vi "Begin.vi"(8 "error in":errorcluster) -> (0 "error out":errorcluster)   [LabVIEW 2015]
doc: "Called before other user functions, this VI is expected to open initial I/O refnums, load in file data, and do all program initialization. Notice that the <B>error out</B> terminal is simply used for data flow. Wiring it to other structures or subVIs ensures that this VI runs first."
uses:
  <vilib>/Rock Robotics/WPI/DriverStation/WPI_DriverStationRobotMode2.ctl
  <vilib>/Rock Robotics/WPI/Joystick/WPI_JoystickDeviceEnum.ctl
  <vilib>/Rock Robotics/WPI/Solenoid/WPI_SolenoidChannel.ctl
  <vilib>/Rock Robotics/SystemInterfaces/DIO/FPGA_DIOPWMChannel.ctl
  <vilib>/Rock Robotics/WPI/SafetyOutput/WPI_SafetyOutputConfigMenu.ctl
  <vilib>/Rock Robotics/SystemInterfaces/DIO/FPGA_DIOChannel.ctl
  Robot Global Data.vi
  <vilib>/Rock Robotics/Network Tables/NT Write String Array.vi
  <vilib>/Rock Robotics/WPI/Solenoid/WPI_SolenoidOpenSingle.vi
  <vilib>/Rock Robotics/WPI/MotorControl/WPI_MotorControlOpen Talon.vi
  <vilib>/Rock Robotics/WPI/MotorControl/WPI_MotorControlOpenCANTalonSRX.vi
  <vilib>/Rock Robotics/WPI/RobotDrive/WPI_RobotDriveOpen4MotorWithCANTalonSRX.vi
  <vilib>/Rock Robotics/WPI/Counter/WPI_CounterDigitalInputToDigitalSource.vi
  <vilib>/Rock Robotics/SystemInterfaces/AI/FPGA_AIGyroChannel.ctl
  <vilib>/Rock Robotics/WPI/MotorControl/WPI_MotorControlOpen Victor.vi
  <vilib>/Rock Robotics/WPI/Gyro/WPI_GyroAnalogOpen.vi
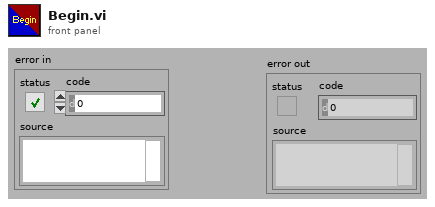
[diagram p1: front panel]
types:
  T1 = typedef "FPGA_DIOChannel.ctl" = enum8{"DIO 0", "DIO 1", "DIO 2", "DIO 3", "DIO 4", "DIO 5", "DIO 6", "DIO 7", "DIO 8", "DIO 9", "DIO MXP 0", "DIO MXP 1", "DIO MXP 2", "DIO MXP 3", "DIO MXP 4", "DIO MXP 5", "DIO MXP 6", "DIO MXP 7", "DIO MXP 8", "DIO MXP 9", "DIO MXP 10", "DIO MXP 11", "DIO MXP 12", "DIO MXP 13", "DIO MXP 14", "DIO MXP 15", "Invalid"}
  T2 = typedef "WPI_SafetyOutputConfigMenu.ctl" = enum16{"Enable", "Disable"}
  T3 = typedef "WPI_SolenoidChannel.ctl" = enum8{"Solenoid 0", "Solenoid 1", "Solenoid 2", "Solenoid 3", "Solenoid 4", "Solenoid 5", "Solenoid 6", "Solenoid 7", "Invalid"}
  T4 = typedef "FPGA_DIOPWMChannel.ctl" = enum8{"PWM 0", "PWM 1", "PWM 2", "PWM 3", "PWM 4", "PWM 5", "PWM 6", "PWM 7", "PWM 8", "PWM 9", "PWM MXP 0", "PWM MXP 1", "PWM MXP 2", "PWM MXP 3", "PWM MXP 4", "PWM MXP 5", "PWM MXP 6", "PWM MXP 7", "PWM MXP 8", "PWM MXP 9", "Invalid"}
  T5 = typedef "WPI_JoystickDeviceEnum.ctl" = enum16{"USB 0", "USB 1", "USB 2", "USB 3", "USB 4", "USB 5"}
  T6 = typedef "WPI_DriverStationRobotMode2.ctl" = enum16{"Autonomous Disabled", "Autonomous Enabled", "Teleop Disabled", "Teleop Enabled", "Disconnected", "Finish", "Test Disabled", "Test Enabled", "Emergency Stopped"}
  T7 = typedef "WPI_DigitalInputDevRef.ctl" = cluster{"DevStatus":errorcluster, "DIO Channel":T1}
  T8 = typedef "FPGA_CounterEncoderSourceConvertionLVSourceType.ctl" = cluster{"DevStatus":errorcluster, "AnalogTriggerMode?":bool, "DigitalMode":cluster{"DIO Channel":T9}, "AnalogTriggerMode":cluster{"AnalogTriggerIndex":T10, "OutputType":T11}}
  T9 = typedef "FPGA_DIODigitalSourceChannel.ctl" = enum8{"DIO 0", "DIO 1", "DIO 2", "DIO 3", "DIO 4", "DIO 5", "DIO 6", "DIO 7", "DIO 8", "DIO 9", "DIO MXP 0", "DIO MXP 1", "DIO MXP 2", "DIO MXP 3", "DIO MXP 4", "DIO MXP 5", "DIO MXP 6", "DIO MXP 7", "DIO MXP 8", "DIO MXP 9", "DIO MXP 10", "DIO MXP 11", "DIO MXP 12", "DIO MXP 13", "DIO MXP 14", "DIO MXP 15", "Disabled"}
  T10 = typedef "FPGA_AnalogTriggerIndex.ctl" = enum8{"Trig 0", "Trig 1", "Trig 2", "Trig 3", "Trig 4", "Trig 5", "Trig 6", "Trig 7", "Invalid"}
  T11 = typedef "FPGA_AnalogTriggerOutType.ctl" = enum16{"InWindow", "TriggerState", "Rising", "Falling"}
  T12 = typedef "WPI_EncoderDevRef.ctl" = cluster{"DevStatus":errorcluster, "EncoderIndex":T13, "CounterIndex":T14, "DistancePerCount":dbl, "Decoding Type":T15}
  T13 = typedef "FPGA_EncoderIdx.ctl" = enum8{"Enc 0", "Enc 1", "Enc 2", "Enc 3", "Enc 4", "Enc 5", "Enc 6", "Enc 7", "Invalid"}
  T14 = typedef "FPGA_CounterCtrSystemIndex.ctl" = enum8{"Ctr 0", "Ctr 1", "Ctr 2", "Ctr 3", "Ctr 4", "Ctr 5", "Ctr 6", "Ctr 7", "Invalid"}
  T15 = typedef "WPI_EncoderType.ctl" = enum16{"1x", "2x", "4x"}
  T16 = typedef "WPI_JoystickDevRef.ctl" = cluster{"Device":T5}
  T17 = typedef "WPI_SolenoidDevRef.ctl" = cluster{"DevStatus":errorcluster, "Pneumatics Control Module":u8, "Forward Solenoid Channel":T3, "Reverse Solenoid Channel":T3}
  T18 = typedef "WPI_MotorControlDeviceRef.ctl" = cluster{"DeviceStatus":errorcluster, "Type":T19, "PWM":cluster{"PWM Channel":T4, "DeadBand":T20}, "CAN":cluster{"Device Number":u8, "Control Mode":T21, "Semaphore":T22, "Max Vout":dbl, "TalonSRX Control Mode":T23}, "Invert":bool}
  T19 = typedef "WPI_MotorControlType.ctl" = enum16{"PWM", "CAN", "CANTalonSRX"}
  T20 = typedef "WPI_PWMDeadband.ctl" = cluster{"Name":string, "maxPositivePwm":i32, "minPositivePwm":i32, "centerPwm":i32, "maxNegativePwm":i32, "minNegativePwm":i32, "angularRange":u16}
  T21 = typedef "WPI_CANJaguar_ControlMode.ctl" = enum8{"Percent VBus", "Current", "Speed", "Position", "Voltage"}
  T22 = typedef "Semaphore RefNum" = refnum<k1>
  T23 = typedef "WPI_CANTalonSRX_APIControlMode.ctl" = enum8{"Percent VBus", "Speed", "Position", "Slave", "Unchanged / Invalid", "Voltage Compensation", "Current", "Motion Profile"}
  T24 = typedef "FPGA_AIGyroChannel.ctl" = enum8{"AI 0", "AI 1", "Invalid"}
  T25 = typedef "WPI_GyroDevRef.ctl" = cluster{"DevStatus":errorcluster, "Analog Channel":T26, "Offset":dbl, "Gain (VoltsPerDegree/Second)":dbl, "Gyro Type":enum16{"Analog", "XRS450"}, "Handle":i32, "SPI Bus":T27, "Device Found":bool, "Sample Rate":dbl, "Calibrate On Open":bool}
  T26 = typedef "FPGA_AIChannel.ctl" = enum8{"AI 0", "AI 1", "AI 2", "AI 3", "AI MXP 0", "AI MXP 1", "AI MXP 2", "AI MXP 3", "Invalid"}
  T27 = typedef "spi_bus.ctl" = enum16{"SPI On-Board, CS0", "SPI On-Board, CS1", "SPI On-Board, CS2", "SPI On-Board, CS3", "SPI MXP", "Invalid"}
  T28 = typedef "WPI_RobotDriveDevRef.ctl" = cluster{"DevStatus":errorcluster, "Motors[]":T18[], "Square Inputs":bool, "Max Output":dbl}
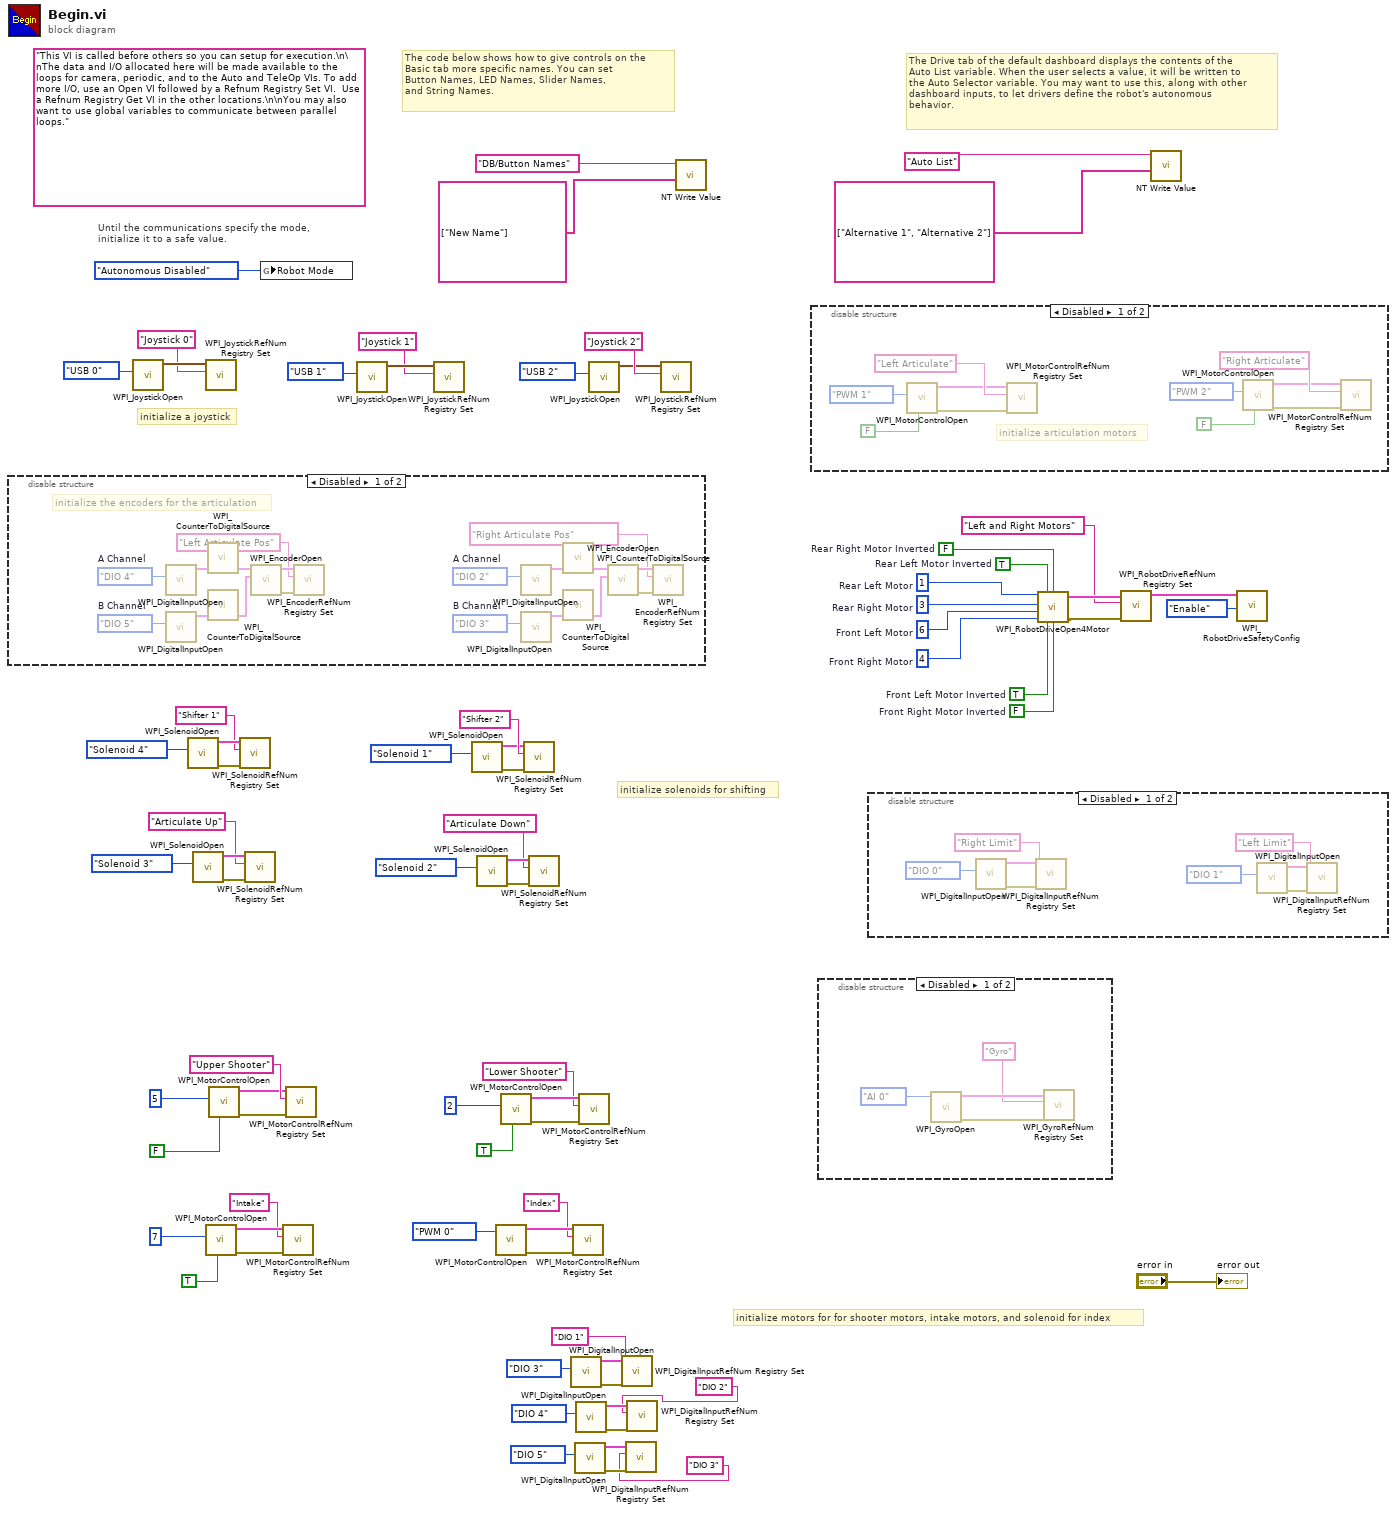
[diagram p0: block diagram]
diagram:
  w25 = u8 4  # Front Right Motor
  w24 = u8 3  # Rear Right Motor
  w23 = u8 6  # Front Left Motor
  w22 = u8 1  # Rear Left Motor
  w21 = TRUE  # Rear Left Motor Inverted
  w20 = FALSE  # Rear Right Motor Inverted
  w19 = FALSE  # Front Right Motor Inverted
  w18 = TRUE  # Front Left Motor Inverted
  (unwired) "This VI is called before others so you can setup for execution.\n\nThe data and I/O allocated here will be made available to the loops for camera, periodic, and to the Auto and TeleOp VIs. To add more I/O, use an Open VI followed by a Refnum Registry Set VI.  Use a Refnum Registry Get VI in the other locations.\n\nYou may also want to use global variables to communicate between parallel loops."
  # "initialize solenoids for shifting"
  # "initialize a joystick"
  # "initialize motors for for shooter motors, intake motors, and solenoid for index"
  # "The Drive tab of the default dashboard displays the contents of the\nAuto List variable. When the user selects a value, it will be written to\nthe Auto Selector variable. You may want to use this, along with other\ndashboard inputs, to let drivers define the robot's autonomous\nbehavior."
  # "The code below shows how to give controls on the\nBasic tab more specific names. You can set\nButton Names, LED Names, Slider Names,\nand String Names."
  # "Until the communications specify the mode,\ninitialize it to a safe value."
  n1 = disable-structure shown="Disabled" {
    frame Disabled {
      w77 = FPGA_DIOChannel."DIO 5"  # B Channel
      w78 = FPGA_DIOChannel."DIO 4"  # A Channel
      w93 = FPGA_DIOChannel."DIO 3"  # B Channel
      w92 = FPGA_DIOChannel."DIO 2"  # A Channel
      # "initialize the encoders for the articulation"
      n2 = call <vilib>:"WPI_DigitalInputOpen.vi"("DIO Channel"=w78) -> ("DigitalInputDevRef"=w81:T7)  [unwired: 1 in, 9 out]
      n3 = call <vilib>:"WPI_DigitalInputOpen.vi"("DIO Channel"=w77) -> ("DigitalInputDevRef"=w80:T7)  [unwired: 1 in, 9 out]
      n4 = call-poly <vilib>:"WPI_CounterToDigitalSource.vi"("DigitalInputDevRef"=w81) -> ("Digital Source"=w82:T8)  [unwired: 6 out]
      n5 = call-poly <vilib>:"WPI_CounterToDigitalSource.vi"("DigitalInputDevRef"=w80) -> ("Digital Source"=w79:T8)  [unwired: 6 out]
      n6 = call <vilib>:"WPI_EncoderOpen.vi"("BSource"=w79, "ASource"=w82) -> ("error out"=w83:errorcluster, "EncoderDevRef"=w84:T12)  [unwired: 6 in, 2 out]
      n7 = call <vilib>:"WPI_EncoderRefNum Registry Set.vi"("error in (no error)"=w83, "refnum name"="Left Articulate Pos", "EncoderDevRef"=w84) -> ()  [unwired: 7 in, 2 out]
      n8 = call <vilib>:"WPI_DigitalInputOpen.vi"("DIO Channel"=w92) -> ("DigitalInputDevRef"=w89:T7)  [unwired: 1 in, 9 out]
      n9 = call <vilib>:"WPI_DigitalInputOpen.vi"("DIO Channel"=w93) -> ("DigitalInputDevRef"=w90:T7)  [unwired: 1 in, 9 out]
      n10 = call-poly <vilib>:"WPI_CounterToDigitalSource.vi"("DigitalInputDevRef"=w89) -> ("Digital Source"=w88:T8)  [unwired: 6 out]
      n11 = call-poly <vilib>:"WPI_CounterToDigitalSource.vi"("DigitalInputDevRef"=w90) -> ("Digital Source"=w91:T8)  [unwired: 6 out]
      n12 = call <vilib>:"WPI_EncoderOpen.vi"("BSource"=w91, "ASource"=w88) -> ("error out"=w87:errorcluster, "EncoderDevRef"=w86:T12)  [unwired: 6 in, 2 out]
      n13 = call <vilib>:"WPI_EncoderRefNum Registry Set.vi"("error in (no error)"=w87, "refnum name"="Right Articulate Pos", "EncoderDevRef"=w86) -> ()  [unwired: 7 in, 2 out]
    }
    frame Enabled {
    }
  }
  n14 = call <vilib>:"WPI_JoystickOpen.vi"("JoystickDevice"=WPI_JoystickDeviceEnum."USB 0") -> ("JoystickDevRef"=w68:T16)  [unwired: 10 in]
  n15 = call-poly <vilib>:"WPI_SolenoidOpen.vi"("Solenoid Channel"=WPI_SolenoidChannel."Solenoid 4") -> ("error out"=w60:errorcluster, "SolenoidDevRef"=w59:T17)  [unwired: 9 in]
  n16 = call-poly <vilib>:"WPI_SolenoidOpen.vi"("Solenoid Channel"=WPI_SolenoidChannel."Solenoid 3") -> ("error out"=w43:errorcluster, "SolenoidDevRef"=w44:T17)  [unwired: 9 in]
  n17 = call <vilib>:"WPI_JoystickRefNum Registry Set.vi"("refnum name"="Joystick 0", "JoystickDevRef"=w68) -> ()  [unwired: 8 in, 2 out]
  n18 = call-poly <vilib>:"WPI_MotorControlOpen.vi"("Invert"=TRUE, "Device Number"=u8 7) -> ("error out"=w30:errorcluster, "MotorControlDeviceRef"=w29:T18)  [unwired: 8 in]
  n19 = call-poly <vilib>:"WPI_MotorControlOpen.vi"("Invert"=FALSE, "Device Number"=u8 5) -> ("error out"=w38:errorcluster, "MotorControlDeviceRef"=w39:T18)  [unwired: 8 in]
  n20 = call <vilib>:"WPI_SolenoidRefNum Registry Set.vi"("error in (no error)"=w60, "refnum name"="Shifter 1", "SolenoidDevRef"=w59) -> ()  [unwired: 7 in, 2 out]
  n21 = call <vilib>:"WPI_SolenoidRefNum Registry Set.vi"("error in (no error)"=w43, "refnum name"="Articulate Up", "SolenoidDevRef"=w44) -> ()  [unwired: 7 in, 2 out]
  n22 = global write "Robot Global Data.vi" "Robot Mode"(WPI_DriverStationRobotMode2."Autonomous Disabled" ("Robot Mode")) -> ()
  n23 = call <vilib>:"WPI_MotorControlRefNum Registry Set.vi"("error in (no error)"=w30, "refnum name"="Intake", "MotorControlDevRef"=w29) -> ()  [unwired: 7 in, 2 out]
  n24 = call <vilib>:"WPI_MotorControlRefNum Registry Set.vi"("error in (no error)"=w38, "refnum name"="Upper Shooter", "MotorControlDevRef"=w39) -> ()  [unwired: 7 in, 2 out]
  n25 = call <vilib>:"WPI_JoystickOpen.vi"("JoystickDevice"=WPI_JoystickDeviceEnum."USB 1") -> ("JoystickDevRef"=w65:T16)  [unwired: 10 in]
  n26 = call <vilib>:"WPI_JoystickRefNum Registry Set.vi"("refnum name"="Joystick 1", "JoystickDevRef"=w65) -> ()  [unwired: 8 in, 2 out]
  n27 = call-poly <vilib>:"WPI_SolenoidOpen.vi"("Solenoid Channel"=WPI_SolenoidChannel."Solenoid 1") -> ("error out"=w53:errorcluster, "SolenoidDevRef"=w54:T17)  [unwired: 9 in]
  n28 = call-poly <vilib>:"WPI_SolenoidOpen.vi"("Solenoid Channel"=WPI_SolenoidChannel."Solenoid 2") -> ("error out"=w48:errorcluster, "SolenoidDevRef"=w47:T17)  [unwired: 9 in]
  n29 = call-poly <vilib>:"WPI_MotorControlOpen.vi"("PWM Channel"=FPGA_DIOPWMChannel."PWM 0") -> ("error out"=w52:errorcluster, "MotorControlDeviceRef"=w51:T18)  [unwired: 9 in]
  n30 = call-poly <vilib>:"WPI_MotorControlOpen.vi"("Invert"=TRUE, "Device Number"=u8 2) -> ("error out"=w37:errorcluster, "MotorControlDeviceRef"=w36:T18)  [unwired: 8 in]
  n31 = call <vilib>:"WPI_SolenoidRefNum Registry Set.vi"("error in (no error)"=w53, "refnum name"="Shifter 2", "SolenoidDevRef"=w54) -> ()  [unwired: 7 in, 2 out]
  n32 = call <vilib>:"WPI_SolenoidRefNum Registry Set.vi"("error in (no error)"=w48, "refnum name"="Articulate Down", "SolenoidDevRef"=w47) -> ()  [unwired: 7 in, 2 out]
  n33 = call <vilib>:"WPI_DigitalInputOpen.vi"("DIO Channel"=FPGA_DIOChannel."DIO 3") -> ("error out"=w12:errorcluster, "DigitalInputDevRef"=w11:T7)  [unwired: 9 in]
  n34 = call <vilib>:"WPI_MotorControlRefNum Registry Set.vi"("error in (no error)"=w52, "refnum name"="Index", "MotorControlDevRef"=w51) -> ()  [unwired: 7 in, 2 out]
  n35 = call <vilib>:"WPI_DigitalInputOpen.vi"("DIO Channel"=FPGA_DIOChannel."DIO 5") -> ("error out"=w6:errorcluster, "DigitalInputDevRef"=w5:T7)  [unwired: 9 in]
  n36 = call <vilib>:"WPI_DigitalInputOpen.vi"("DIO Channel"=FPGA_DIOChannel."DIO 4") -> ("error out"=w7:errorcluster, "DigitalInputDevRef"=w8:T7)  [unwired: 9 in]
  n37 = call <vilib>:"WPI_MotorControlRefNum Registry Set.vi"("error in (no error)"=w37, "refnum name"="Lower Shooter", "MotorControlDevRef"=w36) -> ()  [unwired: 7 in, 2 out]
  n38 = call <vilib>:"WPI_JoystickOpen.vi"("JoystickDevice"=WPI_JoystickDeviceEnum."USB 2") -> ("JoystickDevRef"=w62:T16)  [unwired: 10 in]
  n39 = call <vilib>:"WPI_DigitalInputRefNum Registry Set.vi"("error in (no error)"=w12, "refnum name"="DIO 1", "DigitalInputDevRef"=w11) -> ()  [unwired: 7 in, 2 out]
  n40 = call <vilib>:"WPI_DigitalInputRefNum Registry Set.vi"("error in (no error)"=w6, "refnum name"="DIO 3", "DigitalInputDevRef"=w5) -> ()  [unwired: 7 in, 2 out]
  n41 = call <vilib>:"WPI_DigitalInputRefNum Registry Set.vi"("error in (no error)"=w7, "refnum name"="DIO 2", "DigitalInputDevRef"=w8) -> ()  [unwired: 7 in, 2 out]
  n42 = call <vilib>:"WPI_JoystickRefNum Registry Set.vi"("refnum name"="Joystick 2", "JoystickDevRef"=w62) -> ()  [unwired: 8 in, 2 out]
  n43 = call-poly <vilib>:"NT Write Value.vi"("String Array"=string[] ["New Name"], "Name"="DB/Button Names") -> ()  [unwired: 9 in, 1 out]
  n44 = disable-structure shown="Disabled" {
    frame Disabled {
      # "initialize articulation motors"
      n45 = call-poly <vilib>:"WPI_MotorControlOpen.vi"("Invert"=FALSE ("Invert Left"), "PWM Channel"=FPGA_DIOPWMChannel."PWM 1") -> ("error out"=w99:errorcluster, "MotorControlDeviceRef"=w100:T18)  [unwired: 8 in]
      n46 = call <vilib>:"WPI_MotorControlRefNum Registry Set.vi"("error in (no error)"=w99, "refnum name"="Left Articulate", "MotorControlDevRef"=w100) -> ()  [unwired: 7 in, 2 out]
      n47 = call-poly <vilib>:"WPI_MotorControlOpen.vi"("Invert"=FALSE ("Invert Right"), "PWM Channel"=FPGA_DIOPWMChannel."PWM 2") -> ("error out"=w96:errorcluster, "MotorControlDeviceRef"=w97:T18)  [unwired: 8 in]
      n48 = call <vilib>:"WPI_MotorControlRefNum Registry Set.vi"("error in (no error)"=w96, "refnum name"="Right Articulate", "MotorControlDevRef"=w97) -> ()  [unwired: 7 in, 2 out]
    }
    frame Enabled {
    }
  }
  n49 = disable-structure shown="Disabled" {
    frame Disabled {
      n50 = call-poly <vilib>:"WPI_GyroOpen.vi"("Analog Channel"=FPGA_AIGyroChannel."AI 0") -> ("error out"=w106:errorcluster, "GyroDevRef"=w107:T25)  [unwired: 8 in, 1 out]
      n51 = call <vilib>:"WPI_GyroRefNum Registry Set.vi"("error in (no error)"=w106, "refnum name"="Gyro", "GyroDevRef"=w107) -> ()  [unwired: 7 in, 2 out]
    }
    frame Enabled {
    }
  }
  n52 = disable-structure shown="Disabled" {
    frame Disabled {
      n53 = call <vilib>:"WPI_DigitalInputOpen.vi"("DIO Channel"=FPGA_DIOChannel."DIO 0") -> ("error out"=w114:errorcluster, "DigitalInputDevRef"=w113:T7)  [unwired: 9 in]
      n54 = call <vilib>:"WPI_DigitalInputRefNum Registry Set.vi"("error in (no error)"=w114, "refnum name"="Right Limit", "DigitalInputDevRef"=w113) -> ()  [unwired: 7 in, 2 out]
      n55 = call <vilib>:"WPI_DigitalInputOpen.vi"("DIO Channel"=FPGA_DIOChannel."DIO 1") -> ("error out"=w111:errorcluster, "DigitalInputDevRef"=w112:T7)  [unwired: 9 in]
      n56 = call <vilib>:"WPI_DigitalInputRefNum Registry Set.vi"("error in (no error)"=w111, "refnum name"="Left Limit", "DigitalInputDevRef"=w112) -> ()  [unwired: 7 in, 2 out]
    }
    frame Enabled {
    }
  }
  n57 = call-poly <vilib>:"WPI_RobotDriveOpen4Motor.vi"("Rear Left Motor"=w22, "Rear Left Motor Inverted"=w21, "Rear Right Motor Inverted"=w20, "Rear Right Motor"=w24, "Front Left Motor"=w23, "Front Right Motor"=w25, "Front Left Motor Inverted"=w18, "Front Right Motor Inverted"=w19) -> ("RobotDriveDevRef"=w16:T28, "error out"=w17:errorcluster)  [unwired: 6 in]
  n58 = call <vilib>:"WPI_RobotDriveRefNum Registry Set.vi"("error in (no error)"=w17, "refnum name"="Left and Right Motors", "RobotDriveDevRef"=w16) -> ("RobotDriveDevRef"=w14:T28)  [unwired: 1 in, 7 out]
  n59 = call-poly <vilib>:"NT Write Value.vi"("String Array"=string[] ["Alternative 1", "Alternative 2"], "Name"="Auto List") -> ()  [unwired: 9 in, 1 out]
  n60 = call <vilib>:"WPI_RobotDriveSafetyConfig.vi"("mode"=WPI_SafetyOutputConfigMenu."Enable", "RobotDriveDevRef"=w14) -> ()  [unwired: 8 in, 2 out]
  "error out" <- "error in"
